vi "trim braces.vi"(0 "string":string) -> (1 "braces?":bool, 2 "trimmed string":string)   [LabVIEW 2024, in "controls manager.lvlib"]
uses:
  controls manager.lvlib
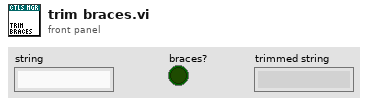
[diagram p1: front panel]
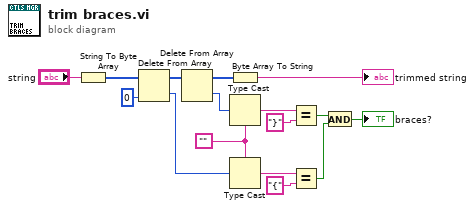
[diagram p0: block diagram]
diagram:
  w10 = ""
  n1 = String To Byte Array(string="string") -> (unsigned byte array=w16:u8[])
  n2 = Delete From Array(array=w16, index=0) -> (deleted portion=w12:u8, array with subset deleted=w15:u8[])  [unwired: 1 in]
  n3 = Delete From Array(array=w15) -> (deleted portion=w11:u8, array with subset deleted=w14:u8[])  [unwired: 2 in]
  n4 = Byte Array To String(unsigned byte array=w14) -> (string=→"trimmed string":string)
  n5 = Type Cast(type=w10, x=w11) -> (*(type *) &x=w7:string)
  n6 = Type Cast(type=w10, x=w12) -> (*(type *) &x=w5:string)
  n7 = Equal?(x=w7, y="}") -> (x = y?=w3:bool)
  n8 = Equal?(x=w5, y="{") -> (x = y?=w2:bool)
  n9 = And(x=w3, y=w2) -> (x .and. y?=→"braces?":bool)
